vi "TWO_button_dialog.vi"(8 "error in (no error)":errorcluster, 11 "message":string) -> (0 "error out":errorcluster, 3 "si/no":bool)   [LabVIEW 2019, in "SHARED VI'S.lvlib"]
uses:
  SHARED VI'S.lvlib
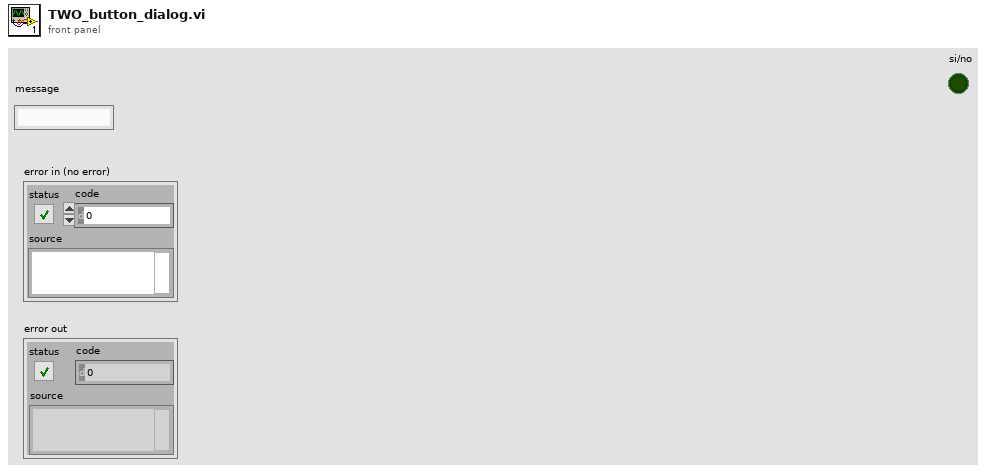
[diagram p1: front panel]
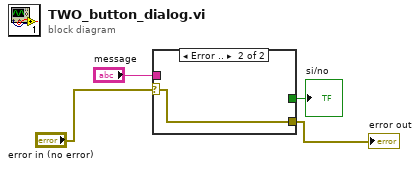
[diagram p0: block diagram]
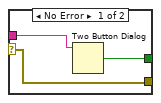
[diagram p2: hidden frame]
diagram:
  n1 = case shown="Error .." "error in (no error)" {
    selector: "error in (no error)" -> [w6 w8]
    tunnel: "message" -> [w7 _]
    tunnel: [w6 w8] -> w2
    tunnel: [w5 _] -> w1
    frame No Error {
      n2 = Two Button Dialog(message=w7) -> (T button?=w5:bool)  [unwired: 2 in]
    }
    frame Error {
    }
  }
  "error out" <- w2
  "si/no" <- w1
